vi "User_Event_Abort.vi"(8 "Error In":errorcluster, 11 "Action":T1) -> (0 "Error Out":errorcluster, 3 "Abort All":refnum<user-event>)   [LabVIEW 2020]
uses:
  Controls/UEA_Action.ctl
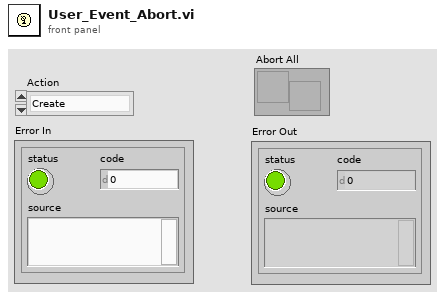
[diagram p1: front panel]
types:
  T1 = typedef "UEA_Action.ctl" = enum16{"Create", "Get", "Destroy"}
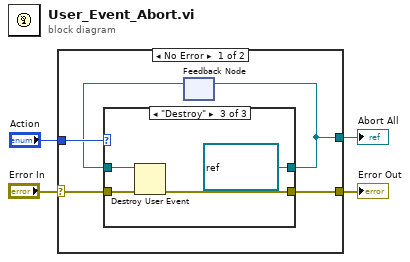
[diagram p0: block diagram]
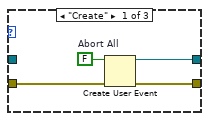
[diagram p2: hidden frame]
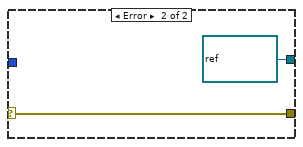
[diagram p4: hidden frame]
diagram:
  n1 = case shown="No Error" "Error In" {
    selector: "Error In" -> [w5 w21]
    tunnel: "Action" -> [w9 _]
    tunnel: [w8 w21] -> w3
    tunnel: [w7 refnum<user-event> refnum ("Abort All")] -> w2
    frame No Error {
      n2 = feedback #1() -> (w6:refnum<user-event>)  [unwired: 1 in]
      n3 = case shown="\"Destroy\"" w9 {
        tunnel: [w12 w15 refnum<user-event> refnum ("Abort All")] -> w7
        tunnel: w5 -> [w11 w14 w19]
        tunnel: [w10 w14 w16] -> w8
        tunnel: w6 -> [_ w15 w17]
        frame "Create" {
          w13 = FALSE  # Abort All
          n4 = Create User Event(user event datatype=w13, error in=w11) -> (user event=w12:refnum<user-event>, error out=w10:errorcluster)
        }
        frame "Get", Default {
        }
        frame "Destroy" {
          n5 = Destroy User Event(user event=w17, error in=w19) -> (error out=w16:errorcluster)
        }
      }
      n6 = feedback-in #1(w7) -> ()
    }
    frame Error {
    }
  }
  "Error Out" <- w3
  "Abort All" <- w2
